vi "DBM Var to Data.vi"(8 "에러 입력":errorcluster caption="에러 입력(에러 없음)", 11 "값":variant) -> (0 "에러 출력":errorcluster, 3 "데이터":T1)   [LabVIEW 2020]
uses:
  Controls/Clst_DBM data.ctl
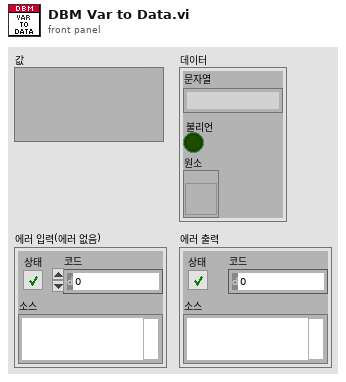
[diagram p1: front panel]
types:
  T1 = typedef "Clst_DBM data.ctl" = cluster{"문자열":string, "불리언":bool, "원소":refnum<vi>}
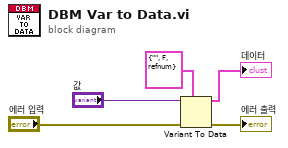
[diagram p0: block diagram]
diagram:
  n1 = Variant To Data(error in="에러 입력", type=T1 {"문자열"="", "불리언"=FALSE, "원소"=refnum} ("데이터"), Variant="값") -> (data=→"데이터":T1, error out=→"에러 출력":errorcluster)
